vi "solar_excel Workbook Open.vi"(8 "error in (no error)":errorcluster, 10 "Excel Workbook (*.xlsx)":path, 11 "Excel App":T1) -> (0 "error out":errorcluster, 3 "Excel Workbook":T2)   [LabVIEW 2018]
doc: "This opens a Workbook reference specified by the <b>Excel Workbook</b> path."
uses:
  solar_excel_ctl Workbook.ctl
  solar_excel_ctl TSV.ctl
  solar_excel_ctl App.ctl
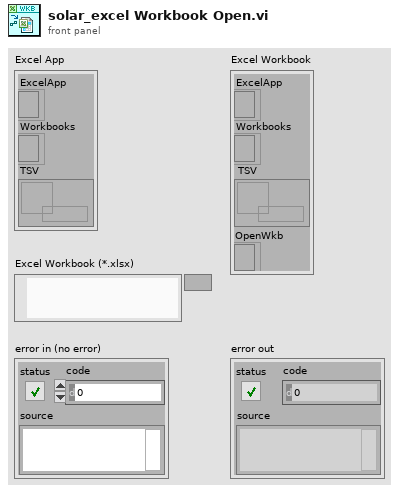
[diagram p1: front panel]
types:
  T1 = typedef "solar_excel_ctl App.ctl" = cluster{"ExcelApp":refnum<k7>, "Workbooks":refnum<k7>, "TSV":refnum<queue>}
  T2 = typedef "solar_excel_ctl Workbook.ctl" = cluster{"ExcelApp":refnum<k7>, "Workbooks":refnum<k7>, "TSV":refnum<queue>, "OpenWkb":refnum<k7>}
  T3 = typedef "solar_excel_ctl TSV.ctl" = cluster{"Path":path, "Dirty":bool, "ActiveSheet":u8, "Worksheets":string[], "Worksheet Cells":cluster{"Cells":string[][]}[]}
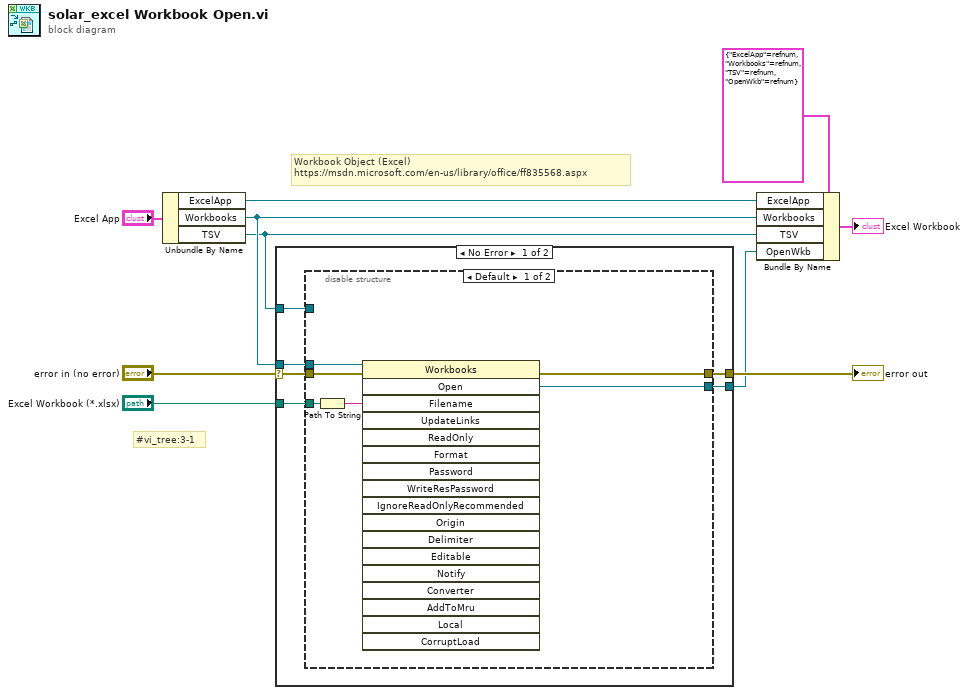
[diagram p0: block diagram]
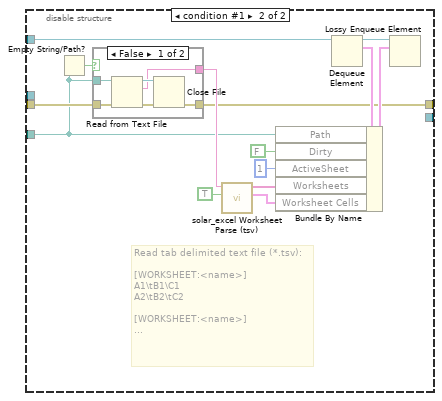
[diagram p2: hidden frame]
diagram:
  # "#vi_tree:3-1"
  # "Workbook Object (Excel)\nhttps://msdn.microsoft.com/en-us/library/office/ff835568.aspx"
  n1 = Unbundle By Name("Excel App") -> ("ExcelApp"=w4:refnum<k7>, "Workbooks"=w3:refnum<k7>, "TSV"=w1:refnum<queue>)
  n2 = case shown="No Error" "error in (no error)" {
    selector: "error in (no error)" -> [w16 w44]
    tunnel: [w13 w44] -> w10
    tunnel: w3 -> [w15 _]
    tunnel: "Excel Workbook (*.xlsx)" -> [w14 _]
    tunnel: [w12 _] -> w2
    tunnel: w1 -> [w11 _]
    frame No Error {
      n3 = disable-structure shown="Default" {
        disable-tunnel: w16 -> [w22 w29]
        disable-tunnel: w15 -> [w21 _]
        disable-tunnel: w14 -> [w20 w28]
        disable-tunnel: [w18 w24] -> w13
        disable-tunnel: [w17 _] -> w12
        disable-tunnel: w11 -> [_ w36]
        frame condition #0 (active) {
          n4 = Path To String(path=w20) -> (string=w19:string)
          n5 = invoke class="Workbooks" method="Open"(reference=w21, error in=w22, "Filename"=w19) -> (error out=w18:errorcluster, "Open"=w17:refnum<k7>)  [unwired: 15 in, 16 out]
        }
        frame condition #1 {
          # "Read tab delimited text file (*.tsv):\n\n[WORKSHEET:<name>]\nA1\\tB1\\C1\nA2\\tB2\\tC2\n\n[WORKSHEET:<name>]\n..."
          n6 = Empty String/Path?(string/path=w28) -> (empty?=w31:bool)
          n7 = case shown="False" w31 {
            tunnel: w28 -> [w41 _]
            tunnel: [w42 w43] -> w24
            tunnel: [w38 _] -> w30
            tunnel: w29 -> [w37 w43]
            frame False {
              n8 = Read from Text File(file (use dialog)=w41, error in=w37) -> (refnum out=w39:refnum<file>, text=w38:string, error out=w40:errorcluster)  [unwired: 2 in, 1 out]
              n9 = Close File(refnum=w39, error in=w40) -> (error out=w42:errorcluster)  [unwired: 1 out]
            }
            frame True {
            }
          }
          n10 = call "solar_excel Worksheet Parse (tsv).vi"("Remove Quotes? (F)"=TRUE, "Tab Delimited String"=w30) -> ("Worksheets Cells"=w26:cluster{"Cells":string[][]}[], "Worksheets"=w27:string[])  [unwired: 8 in]
          n11 = Dequeue Element(queue=w36) -> (queue out=w34:refnum<queue>, element=w35:T3)  [unwired: 2 in, 2 out]
          n12 = Bundle By Name(cluster=w35, "Path"=w28, "Dirty"=FALSE, "ActiveSheet"=u8 1, "Worksheets"=w27, "Worksheet Cells"=w26) -> (w33:T3)
          n13 = Lossy Enqueue Element(queue=w34, element=w33) -> ()  [unwired: 1 in, 4 out]
        }
      }
    }
    frame Error {
    }
  }
  "error out" <- w10
  n14 = Bundle By Name(cluster=T2 {"ExcelApp"=refnum, "Workbooks"=refnum, "TSV"=refnum, "OpenWkb"=refnum} ("Excel Workbook"), "ExcelApp"=w4, "Workbooks"=w3, "TSV"=w1, "OpenWkb"=w2) -> (→"Excel Workbook":T2)
